vi "Properties To Ignore.vi"() -> ()   [LabVIEW 2010, in "NI_SE_Front Panel Layout.lvlib"]
uses:
  NI_SE_Front Panel Layout.lvlib
panel:
  in  "Ring Font":string="ring font"
  in  "Label Position":string="label position"
  in  "Label Font":string="label font"
  in  "Caption Position":string="caption position"
  in  "Caption Font":string="caption font"
  in  "Size":string="size"
  in  "Position":string="position"
  in  "Text":string="text"
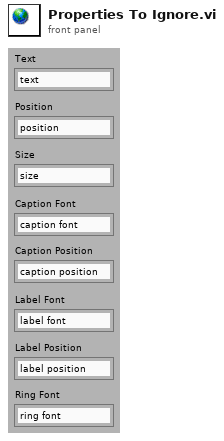
[diagram p1: front panel]
diagram:
